vi "11152 UI.vi"(8 "error in (no error)":errorcluster, 11 "Node Ptr":T1 format="%.0x") -> (0 "error out":errorcluster)   [LabVIEW 2017, in "Modules.lvlib" / "11152.lvclass"]
uses:
  11152.lvclass
  <vilib>/NI Veristand/Custom Device API/Custom Device Item Ref.ctl
  RSI Module/SubPanel Command.ctl
  C:/Users/dbuck/Documents/GitHub/Scan-Engine-Custom-Device-Classes/Source/RemIO Module/RemIO Module.lvclass
  11152.lvclass/11152.ctl
  RemIO Module/RemIO Module.lvclass
  <vilib>/NI Veristand/Custom Device API/Custom Device API.lvlib
  RSI Module/RSI Module.lvclass
panel:
  in  "Input Filter Time":enum16{"500 us", "< 100 us"}(ring)
  in  "SubPanel Event":refnum<user-event>
  in  "Header":cluster{"Section Name":string}={"Section Name"="NI REM-11152 Settings"}
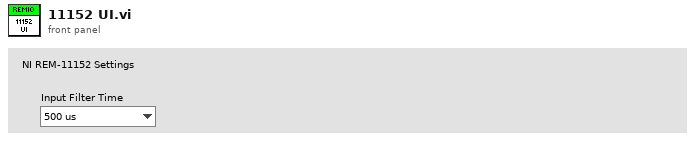
[diagram p1: front panel]
types:
  T1 = typedef "Custom Device API.lvlib/Custom Device Item Ref.ctl" = u64
  T2 = typedef "NI ECAT Remote IO.lvlib/input filter time REM-11152.ctl" = u8
  T3 = typedef "Modules.lvlib/RSI Module.lvclass/SubPanel Command.ctl" = enum16{"Stop"}
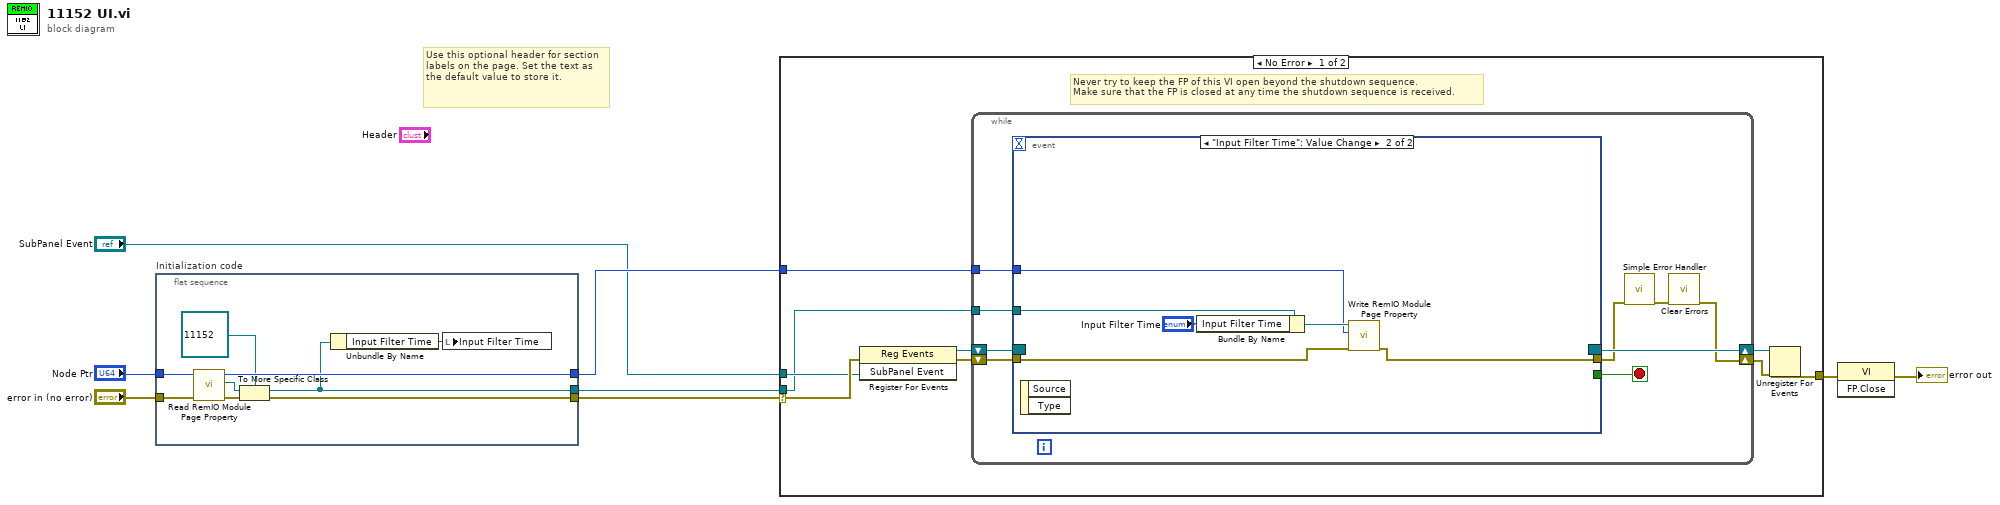
[diagram p0: block diagram]
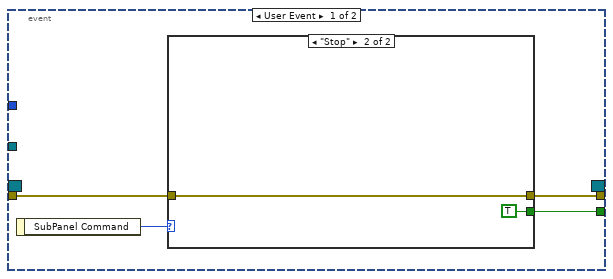
[diagram p2: hidden frame]
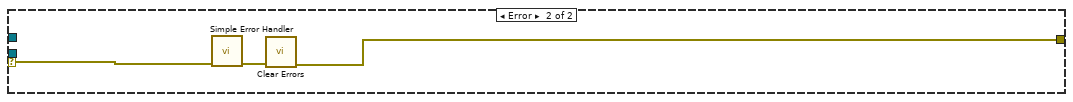
[diagram p4: hidden frame]
diagram:
  # "Use this optional header for section labels on the page. Set the text as the default value to store it."
  n1 = flat-sequence "Initialization code" {
    tunnel: "error in (no error)" -> [w16]
    tunnel: "Node Ptr" -> [w17]
    tunnel: [w11] -> w2
    tunnel: [w15] -> w5
    tunnel: [w10] -> w1
    frame #0 {
      n2 = call "Read RemIO Module Page Property.vi"("error in (no error)"=w16, "Node Ptr In"=w17) -> ("error out"=w14:errorcluster, "RemIO Module"=w13:refnum<class "RemIO Module.lvclass">, "Node Ptr Out"=w15:T1)  [unwired: 7 in]
      n3 = To More Specific Class(target class=refnum<class "11152.lvclass"> refnum ("Modules.lvlib:11152.lvclass"), reference=w13, error in=w14) -> (specific class reference=w10:refnum<class "11152.lvclass">, error out=w11:errorcluster)
      n4 = Unbundle By Name(w10) -> ("Input Filter Time"=w9:T2)
      n5 = local write "Input Filter Time"(w9) -> ()
    }
  }
  n6 = case shown="No Error" w2 {
    selector: w2 -> [w20 w51]
    tunnel: [w24 w49] -> w8
    tunnel: w5 -> [w21 _]
    tunnel: "SubPanel Event" -> [w19 _]
    tunnel: w1 -> [w18 _]
    frame No Error {
      # "Never try to keep the FP of this VI open beyond the shutdown sequence.\nMake sure that the FP is closed at any time the shutdown sequence is received."
      n7 = register-events(error in=w20, w19) -> (reference out=w22:refnum<event-registration>, error out=w23:errorcluster)  [unwired: 1 in]
      n8 = while {
        tunnel: w21 -> [w31]
        shift-right: [w28] -> w25
        shift-left: w23 -> [w34]
        shift-right: [w35] -> w26
        shift-left: w22 -> [w33]
        tunnel: w18 -> [w27]
        stop <- w32 stop-if-true
        n9 = event shown="[1] \"Input Filter Time\": Value Change" {
          selector: w33 -> [_ _]
          dyn-events: [_ _] -> w35
          timeout: _ -> [_ _]
          tunnel: w34 -> [w38 w44]
          tunnel: [w36 _] -> w32
          tunnel: [w37 w43] -> w30
          tunnel: w31 -> [_ w45]
          tunnel: w27 -> [_ w48]
          event User Event {
            n10 = event-data() -> ("SubPanel Command"=w39:T3)  [unwired: 1 out]
            n11 = case shown="\"Stop\"" w39 {
              tunnel: w38 -> [w40 w41]
              tunnel: [w40 w41] -> w37
              tunnel: [_ TRUE] -> w36
              frame Default {
              }
              frame "Stop" {
              }
            }
          }
          event "Input Filter Time": Value Change {
            n12 = event-data() -> ()  [unwired: 3 out]
            n13 = Bundle By Name(cluster=w48, "Input Filter Time"="Input Filter Time") -> (w46:refnum<class "11152.lvclass">)
            n14 = call "Write RemIO Module Page Property.vi"("error in (no error)"=w44, "Node Ptr In"=w45, "RemIO Module"=w46) -> ("error out"=w43:errorcluster)  [unwired: 6 in, 2 out]
          }
        }
        n15 = call <vilib>:"Simple Error Handler.vi"("error in (no error)"=w30) -> ("error out"=w29:errorcluster)  [unwired: 1 in, 7 out]
        n16 = call <vilib>:"Clear Errors.vi"("error in (no error)"=w29) -> ("error out"=w28:errorcluster)  [unwired: 1 in, 5 out]
      }
      n17 = Unregister For Events(event registration refnum=w26, error in=w25) -> (error out=w24:errorcluster)
    }
    frame Error {
      n18 = call <vilib>:"Simple Error Handler.vi"("error in (no error)"=w51) -> ("error out"=w50:errorcluster)  [unwired: 1 in, 7 out]
      n19 = call <vilib>:"Clear Errors.vi"("error in (no error)"=w50) -> ("error out"=w49:errorcluster)  [unwired: 1 in, 5 out]
    }
  }
  n20 = invoke class="VI" method="FP.Close"(error in=w8) -> (error out=→"error out":errorcluster)  [unwired: 2 in, 2 out]
